vi "JSON Field Type.vi"(11 "JSON String":string) -> (3 "JSON Item Type":T1=enum."null")   [LabVIEW 2020, in "JSON.lvlib"]
uses:
  JSON.lvlib
  JSON Item Type.ctl
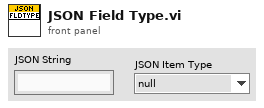
[diagram p1: front panel]
types:
  T1 = typedef "JSON.lvlib/JSON Item Type.ctl" = enum16{"unknown", "null", "Array", "Object", "String", "Number", "Boolean"}
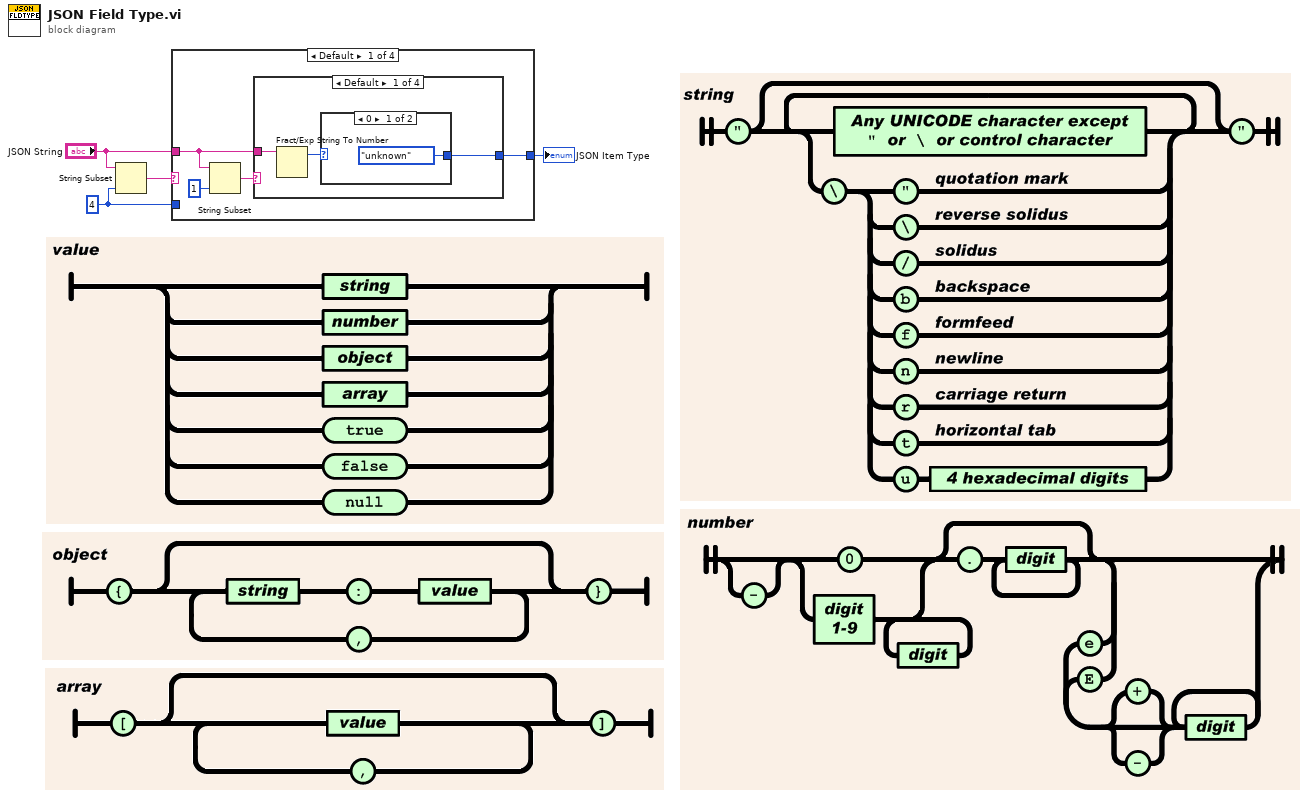
[diagram p0: block diagram]
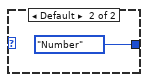
[diagram p2: hidden frame]
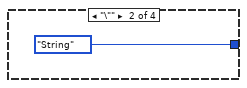
[diagram p3: hidden frame]
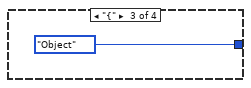
[diagram p4: hidden frame]
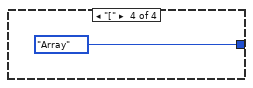
[diagram p5: hidden frame]
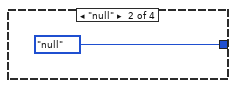
[diagram p6: hidden frame]
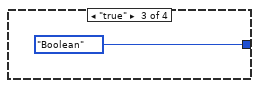
[diagram p7: hidden frame]
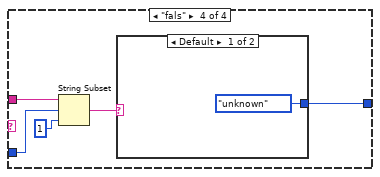
[diagram p8: hidden frame]
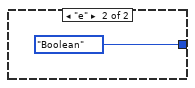
[diagram p9: hidden frame]
diagram:
  w1 = 4 ("length (rest)")
  n1 = String Subset(string="JSON String", length (rest)=w1) -> (substring=w3:string)  [unwired: 1 in]
  n2 = case shown="Default" w3 {
    tunnel: [w5 JSON_Item_Type."null" ("JSON Item Type") JSON_Item_Type."Boolean" ("JSON Item Type") w19] -> w4
    tunnel: "JSON String" -> [w6 _ _ w23]
    tunnel: w1 -> [_ _ _ w22]
    frame Default {
      n3 = String Subset(string=w6, length (rest)=1 ("length (rest)")) -> (substring=w7:string)  [unwired: 1 in]
      n4 = case shown="Default" w7 {
        tunnel: w6 -> [w10 _ _ _]
        tunnel: [w11 JSON_Item_Type."String" ("JSON Item Type") JSON_Item_Type."Object" ("JSON Item Type") JSON_Item_Type."Array" ("JSON Item Type")] -> w5
        frame Default {
          n5 = Fract/Exp String To Number(string=w10) -> (offset past number=w9:i32)  [unwired: 3 in, 1 out]
          n6 = case shown="0" w9 {
            tunnel: [JSON_Item_Type."unknown" ("JSON Item Type") JSON_Item_Type."Number" ("JSON Item Type")] -> w11
            frame 0 {
            }
            frame Default {
            }
          }
        }
        frame "\"" {
        }
        frame "{" {
        }
        frame "[" {
        }
      }
    }
    frame "null" {
    }
    frame "true" {
    }
    frame "fals" {
      n7 = String Subset(string=w23, offset (0)=w22, length (rest)=1 ("length (rest)")) -> (substring=w20:string)
      n8 = case shown="Default" w20 {
        tunnel: [JSON_Item_Type."unknown" ("JSON Item Type") JSON_Item_Type."Boolean" ("JSON Item Type")] -> w19
        frame Default {
        }
        frame "e" {
        }
      }
    }
  }
  "JSON Item Type" <- w4
